vi "RSZVB Set Calibration Connector.vi"(4 "Propagation Mode (0: Transverse electric)":i32(ring) items=["Transverse electric", "Waveguide"], 5 "Impedance (0.0)":dbl format="%^.3e", 6 "Relative Permittivity (0.0)":dbl format="%^.3e", 7 "Connector Type (0: Polar)":i32(ring) items=["Polar", "Sexless"], 8 "error in (no error)":errorcluster {"code" format="%.0x"}, 9 "Connector Name":string, 10 "Channel (1)":i32=1, 11 "VISA session":refnum<visa-resource-name>) -> (0 "error out":errorcluster {"code" format="%.0x"}, 3 "dup VISA session":refnum<visa-resource-name>)   [LabVIEW 2011]
doc: "This VI configures the user-defined connector types.\n\nRemote-control command(s):\n[SENSe<Ch>:]CORRection:CONNection '<conn_name>', TEM | WGUide, GENDer | NGENder, <perm_rel>, <imped>"
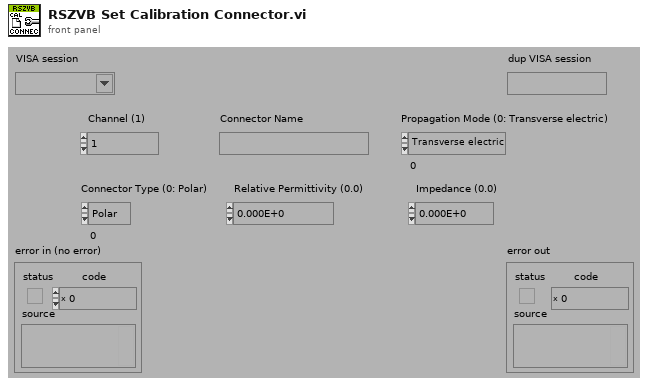
[diagram p1: front panel]
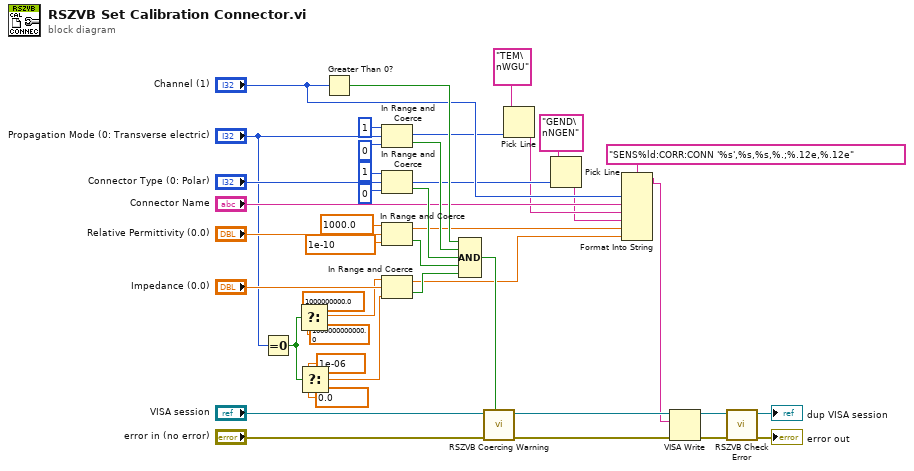
[diagram p0: block diagram]
diagram:
  n1 = Equal To 0?(x="Propagation Mode (0: Transverse electric)") -> (x = 0?=w1:bool)
  n2 = Select(t=1000000000.0 ("lower limit"), s=w1, f=1000000000000.0 ("lower limit")) -> (s? t:f=w2:dbl)
  n3 = Select(t=1e-06 ("lower limit"), s=w1, f=0.0 ("lower limit")) -> (s? t:f=w6:dbl)
  n4 = Greater Than 0?(x="Channel (1)") -> (x > 0?=w25:bool)
  n5 = In Range and Coerce(upper limit=1 ("lower limit"), x="Propagation Mode (0: Transverse electric)", lower limit=0) -> (coerced(x)=w15:i32, In Range?=w24:bool)
  n6 = In Range and Coerce(upper limit=1 ("lower limit"), x="Connector Type (0: Polar)", lower limit=0) -> (coerced(x)=w13:i32, In Range?=w23:bool)
  n7 = In Range and Coerce(upper limit=1000.0, x="Relative Permittivity (0.0)", lower limit=1e-10) -> (coerced(x)=w10:dbl, In Range?=w21:bool)
  n8 = In Range and Coerce(upper limit=w2, x="Impedance (0.0)", lower limit=w6) -> (coerced(x)=w9:dbl, In Range?=w22:bool)
  n9 = Compound Arithmetic op=AND(w25, w24, w23, w21, w22) -> (w37:bool)
  n10 = call "RSZVB Coercing Warning.vi"("In Range?"=w37, "error in (no error)"="error in (no error)", "VISA session"="VISA session") -> ("error out"=w42:errorcluster, "dup VISA session"=w43:refnum<visa-resource-name>)  [unwired: 7 in]
  n11 = Pick Line(multi-line string="TEM\nWGU", line index=w15) -> (output string=w12:string)  [unwired: 1 in]
  n12 = Pick Line(multi-line string="GEND\nNGEN", line index=w13) -> (output string=w11:string)  [unwired: 1 in]
  n13 = Format Into String(format string="SENS%ld:CORR:CONN '%s',%s,%s,%.;%.12e,%.12e", "Channel (1)", "Connector Name", w12, w11, w10, w9) -> (resulting string=w38:string)  [unwired: 2 in, 1 out]
  n14 = VISA Write(VISA resource name=w43, write buffer=w38, error in (no error)=w42) -> (VISA resource name out=w40:refnum<visa-resource-name>, error out=w41:errorcluster)  [unwired: 1 out]
  n15 = call "RSZVB Check Error.vi"("error in (no error)"=w41, "VISA session"=w40) -> ("error out"=→"error out":errorcluster, "dup VISA session"=→"dup VISA session":refnum<visa-resource-name>)  [unwired: 8 in]
